vi "Timer_subVI.vi"(8 "error in (no error)":errorcluster, 11 "Time to elapse (s)":dbl) -> (0 "error out":errorcluster, 2 "timeElapsed?":bool, 3 "Time":dbl)   [LabVIEW 2019]
uses:
  controls/#typedef_Timer_Actions.ctl
panel:
  in  "Timer Action":T1
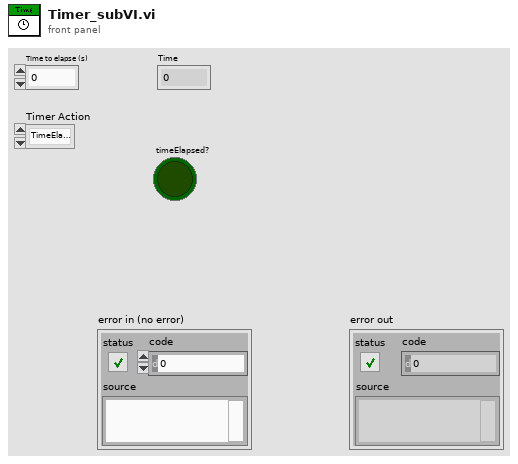
[diagram p1: front panel]
types:
  T1 = typedef "#typedef_Timer_Actions.ctl" = enum16{"TimeElapsed", "reset"}
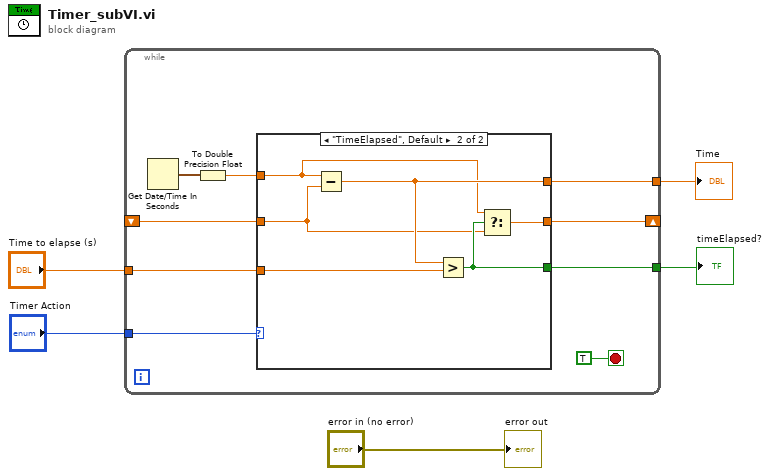
[diagram p0: block diagram]
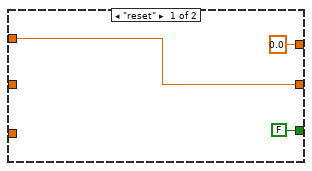
[diagram p2: hidden frame]
diagram:
  n1 = while {
    shift-right: [w9] -> _
    shift-left: _ -> [w11]
    tunnel: "Timer Action" -> [w13]
    tunnel: [w10] -> w4
    tunnel: "Time to elapse (s)" -> [w8]
    tunnel: [w7] -> w5
    stop <- TRUE stop-if-true
    n2 = Get Date/Time In Seconds() -> (seconds since 1Jan1904=w14:timestamp)
    n3 = To Double Precision Float(number=w14) -> (double precision float=w12:dbl)
    n4 = case shown="\"TimeElapsed\", Default" w13 {
      tunnel: w12 -> [w17 w19]
      tunnel: w11 -> [_ w20]
      tunnel: [0.0 w21] -> w10
      tunnel: [w17 w18] -> w9
      tunnel: w8 -> [_ w23]
      tunnel: [FALSE w22] -> w7
      frame "reset" {
      }
      frame "TimeElapsed", Default {
        n5 = Subtract(x=w19, y=w20) -> (x-y=w21:dbl)
        n6 = Greater?(x=w21, y=w23) -> (0:w22:bool)
        n7 = Select(t=w19, s=w22, f=w20) -> (s? t:f=w18:dbl)
      }
    }
  }
  "timeElapsed?" <- w5
  "Time" <- w4
  "error out" <- "error in (no error)"
